vi "_process.vi"(8 "error in (no error)":errorcluster, 11 "_dataProcessing in":refnum<class "_dataProcessing.lvclass">) -> (0 "error out":errorcluster, 3 "_dataProcessing out":refnum<class "_dataProcessing.lvclass">)   [LabVIEW 2019, in "_dataProcessing.lvlib" / "_dataProcessing.lvclass"]
uses:
  _dataProcessing.lvclass
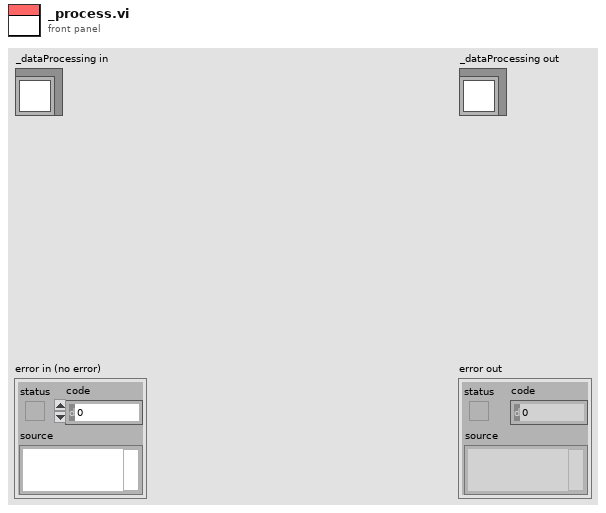
[diagram p1: front panel]
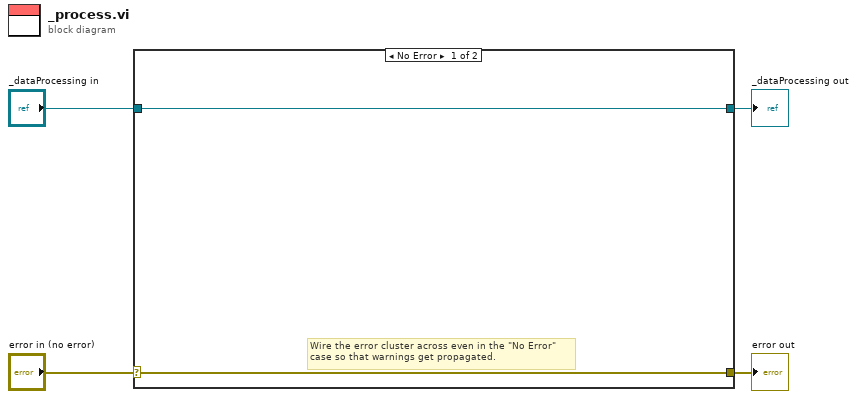
[diagram p0: block diagram]
diagram:
  n1 = case shown="No Error" "error in (no error)" {
    selector: "error in (no error)" -> [w5 w8]
    tunnel: [w5 w8] -> w3
    tunnel: [w6 w7] -> w1
    tunnel: "_dataProcessing in" -> [w6 w7]
    frame No Error {
      # "Wire the error cluster across even in the \"No Error\"\ncase so that warnings get propagated."
    }
    frame Error {
    }
  }
  "error out" <- w3
  "_dataProcessing out" <- w1
